vi "AddToReservedList.vi"(11 "VISA resource":string) -> (1 "Reserved?":bool, 3 "VISA resource out":string)   [LabVIEW 2019]
uses:
  GLOBALS.vi
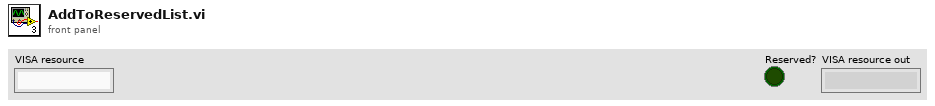
[diagram p1: front panel]
types:
  T1 = typedef "Globals_IO.ctl" = cluster{"Reserved COM ports":cluster{"Port":string, "Reserved By":string, "Time":timestamp}[]}
  T2 = cluster{"Port":string, "Reserved By":string, "Time":timestamp}[]
  T3 = cluster{"VISA resource":string, "spreadsheet string":string, "seconds since 1Jan1904":timestamp}
  T4 = cluster{"VISA resource":string, "spreadsheet string":string, "seconds since 1Jan1904":timestamp}[]
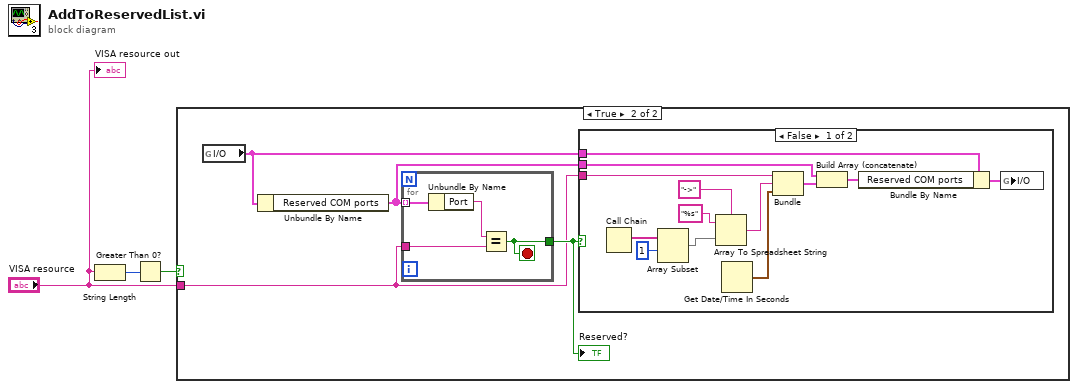
[diagram p0: block diagram]
diagram:
  n1 = String Length(string="VISA resource") -> (length=w2:i32)
  n2 = Greater Than 0?(x=w2) -> (x > 0?=w1:bool)
  n3 = case shown="True" w1 {
    tunnel: "VISA resource" -> [_ w4]
    frame False {
    }
    frame True {
      n4 = global read "Globals.vi" "I/O"() -> (w6:T1)
      n5 = Unbundle By Name(w6) -> ("Reserved COM ports"=w5:T2)
      n6 = for {
        tunnel: w4 -> [w24]
        tunnel: [w23] -> w7
        tunnel: w5 -> [w22] mode=indexing
        stop <- w23 stop-if-true
        n7 = Unbundle By Name(w22) -> ("Port"=w21:string)
        n8 = Equal?(x=w21, y=w24) -> (x = y?=w23:bool)
      }
      "Reserved?" <- w7
      n9 = case shown="False" w7 {
        tunnel: w6 -> [w18 _]
        tunnel: w5 -> [w19 _]
        tunnel: w4 -> [w14 _]
        frame False {
          n10 = Call Chain() -> (call chain=w10:string[])
          n11 = Array Subset(array=w10, index=1) -> (w8:string[])  [unwired: 1 in]
          n12 = Array To Spreadsheet String(delimiter (Tab)="->", array=w8, 3:"%s" ("format string")) -> (spreadsheet string=w13:string)
          n13 = Get Date/Time In Seconds() -> (seconds since 1Jan1904=w12:timestamp)
          n14 = Bundle("VISA resource"=w14, "spreadsheet string"=w13, "seconds since 1Jan1904"=w12) -> (w11:T3)  [unwired: 1 in]
          n15 = Build Array (concatenate)(w19, w11) -> (w17:T4)
          n16 = Bundle By Name(cluster=w18, "Reserved COM ports"=w17) -> (w20:T1)
          n17 = global write "Globals.vi" "I/O"(w20) -> ()
        }
        frame True {
        }
      }
    }
  }
  "VISA resource out" <- "VISA resource"
